vi "Initialize From Settings.vi"(8 "error in (no error)":errorcluster, 10 "settings":cluster{"key":string, "value":string}[](array[cluster]), 11 "Core Transfer Configuration in":refnum<class "Transfer Configuration.lvclass">) -> (0 "error out":errorcluster, 3 "Core Transfer Configuration out":refnum<class "Transfer Configuration.lvclass">)   [LabVIEW 2020, in "DSF Core.lvlib" / "Transfer Configuration.lvclass"]
uses:
  Transfer Configuration.lvclass
  Transfer Configuration.lvclass/Transfer Configuration.ctl
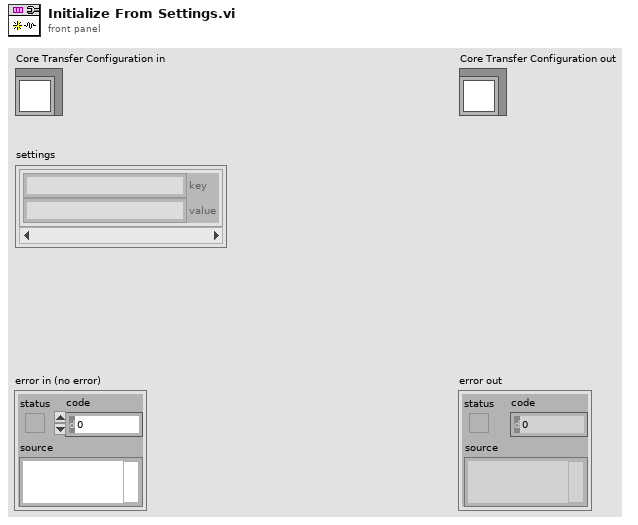
[diagram p1: front panel]
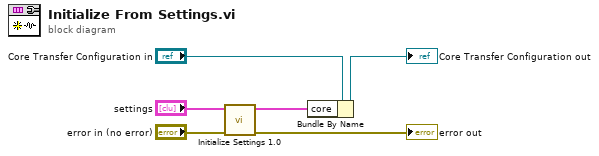
[diagram p0: block diagram]
diagram:
  n1 = call "Initialize Settings 1.0.vi"("error in (no error)"="error in (no error)", "settings 1.0"="settings") -> ("error out"=→"error out":errorcluster, "configuration 1.0"=w2:cluster{"name":string})  [unwired: 8 in]
  n2 = Bundle By Name(cluster="Core Transfer Configuration in", "core"=w2) -> (→"Core Transfer Configuration out":refnum<class "Transfer Configuration.lvclass">)
